vi "Request Events.vi"(8 "error in (no error)":errorcluster, 11 "EventAPI in":refnum<class "EventAPI.lvclass">) -> (0 "error out":errorcluster, 2 "Events":T1[](array[typedef]), 3 "EventAPI out":refnum<class "EventAPI.lvclass">)   [LabVIEW 2020, in "Volatus.lvlib" / "EventAPI.lvclass"]
uses:
  EventAPI.lvclass
  EventAPI.lvclass/EventAPI.ctl
  lv-promises/Promises/Promise/Promise.lvclass
  EventsValue/EventsValue.lvclass
  EventHandler Messages/Request Events Msg/Request Events Msg.lvclass
  lv-promises/Promises/Future/Future.lvclass
  C:/dev/lv20CE/relink/lv-promises/Promises/Value/Value.lvclass
  C:/dev/lv20CE/relink/lv-volatus/Volatus/EventsValue/EventsValue.lvclass
  Event Level.ctl
  Volatus.lvlib
  Event.ctl
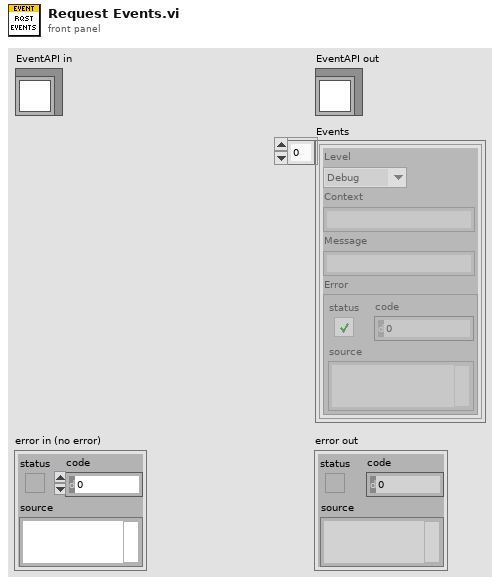
[diagram p1: front panel]
types:
  T1 = typedef "Volatus.lvlib/Event.ctl" = cluster{"Level":T2, "Context":string, "Message":string, "Error":errorcluster}
  T2 = typedef "Volatus.lvlib/Event Level.ctl" = enum16{"Debug", "Info", "Warning", "Error"}
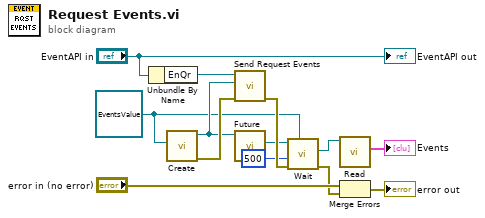
[diagram p0: block diagram]
diagram:
  w5 = refnum<class "EventsValue.lvclass"> refnum ("Volatus:EventsValue.lvclass")
  n1 = Unbundle By Name("EventAPI in") -> ("EnQr"=w9:refnum<class "Message Enqueuer.lvclass">)
  n2 = call "Create.vi"("Result Type"=w5) -> ("error out"=w13:errorcluster, "Promise"=w8:refnum<class "Promise.lvclass">)  [unwired: 9 in]
  n3 = call "Send Request Events.vi"("error in (no error)"=w13, "Promise"=w8, "Message Enqueuer"=w9) -> ("error out"=w12:errorcluster)  [unwired: 7 in, 1 out]
  n4 = call "Future.vi"("Promise in"=w8) -> ("Future"=w7:refnum<class "Future.lvclass">)  [unwired: 9 in, 1 out]
  n5 = call "Wait.vi"("Result Type"=w5, "error in (no error)"=w12, "Timeout mS (-1)"=500, "Future in"=w7) -> ("error out"=w1:errorcluster, "Result"=w4:refnum<class "EventsValue.lvclass">)  [unwired: 6 in]
  n6 = call "Read.vi"("EventsValue in"=w4) -> ("Events"=→"Events":T1[])  [unwired: 10 in]
  n7 = Merge Errors("error in (no error)", w1) -> (→"error out":errorcluster)
  "EventAPI out" <- "EventAPI in"
